vi "InjA-Image-FPGA.vi"() -> ()   [LabVIEW 2015]
uses:
  <vilib>/LabVIEW Targets/FPGA/cRIO/shared/nicrio_ModuleControls/nicrio_cRIO-9871_DataBitsEnum.ctl
  <vilib>/LabVIEW Targets/FPGA/cRIO/shared/nicrio_ModuleControls/nicrio_cRIO-9871_BaudRateEnum.ctl
  <vilib>/LabVIEW Targets/FPGA/cRIO/shared/nicrio_ModuleControls/nicrio_cRIO-9871_ParityEnum.ctl
  <vilib>/LabVIEW Targets/FPGA/cRIO/shared/nicrio_ModuleControls/nicrio_cRIO-9871_StopBitsEnum.ctl
  <vilib>/Platform/TimedLoop/XDataNode/timing_clust.ctl
  <vilib>/Platform/TimedLoop/XDataNode/nitl_modes.ctl
  <vilib>/Platform/TimedLoop/XDataNode/wakeup.ctl
  <vilib>/rvi/FXPMathLib/basic elements/FxpIntAccumulator/subVIs/nifxpmath_IntAccumulator_SimConfig.ctl
  <vilib>/rvi/Emulation/niFpgaGetClockAttributes.vi
  <vilib>/rvi/Emulation/niFpgaSctlEmulationGetInTimedLoop.vi
  <vilib>/rvi/Emulation/niFpgaEmulationReportErrorSimple.vi
  <vilib>/rvi/eio/common/nirviEmuTemplateMethod_errors.vi
  <vilib>/rvi/Emulation/niFpgaCriticalErrorInLSC.vi
  <vilib>/rvi/Analysis/common/codeGenErrors/XNode/niFpgaXNodeCodeGenErrorHandle.vi
  <vilib>/rvi/FXPMathLib/basic elements/FxpIntAccumulator/simVIs/DllFxpIntAccumulator_sub.vi
  <vilib>/rvi/eio/common/nirviEmuTemplatePropertySet_noerrors.vi
  <vilib>/eio/EIOMethodNode/EIOMethodNode.xnode
  <vilib>/eio/EIONode/EIONode.xnode
  <vilib>/rvi/Analysis/measure/dc-rms/XNode/niFpgaDC-RMS.xnode
  <vilib>/Platform/TimedLoop/XDataNode/XDataNode.xnode
  <vilib>/rvi/FXPMathLib/basic elements/FxpIntAccumulator/XNode/nifxpmath_IntAccumulator.xnode
  <vilib>/rvi/FXPMathLib/FxpMul/XNode/nifxpmath_Multiplier.xnode
  <vilib>/eio/EIOPropertyNode/EIOPropertyNode.xnode
  <vilib>/Platform/TimedLoop/XDataNode/XDNodeRunTimeDep.lvlib
  <vilib>/rvi/FXPMathLib/sim/FxpSim.dll
  <vilib>/rvi/eio/common/nirviEmuTemplatePropertyGet_errors.vi
  <vilib>/rvi/eio/common/nirviEmuTemplatePropertyGet_noerrors.vi
  <vilib>/rvi/eio/common/nirviEmuTemplatePropertySet_errors.vi
panel:
  in  "reset":bool
  out "Ion gauge 3":u8[](array[numeric])
  in  "cup set values":bool[](array[boolean])=[FALSE, FALSE, FALSE, FALSE]
  out "cup readbacks":bool[](array[boolean])
  out "1st stage temp(k)":u8[](array[numeric])
  out "2nd stage":u8[](array[numeric])
  out "Time on":u8[](array[numeric])
  out "Pump On":u8[](array[numeric])
  out "Ion gauge 4":u8[](array[numeric])
  out "Convectron 4":u8[](array[numeric])
  out "Convectron 3":u8[](array[numeric])
  out "Analog input":fxp<+/-,26,5>[](array[numeric]) format="%.23g"
  in  "analog output":fxp<+/-,64,32>[](array[numeric])=[0.0, 0.0, 0.0, 0.0, 0.0, 0.0, 0.0]
  in  "magnet ps":u8[](array[numeric])=[0, 0, 0, 0, 0, 0, 0, 0, 0, 0]
  out "error out":errorcluster
  out "magnet field":u8[](array[numeric])
  out "Timed Out":bool
  out "Data":u8
  # "skipped"
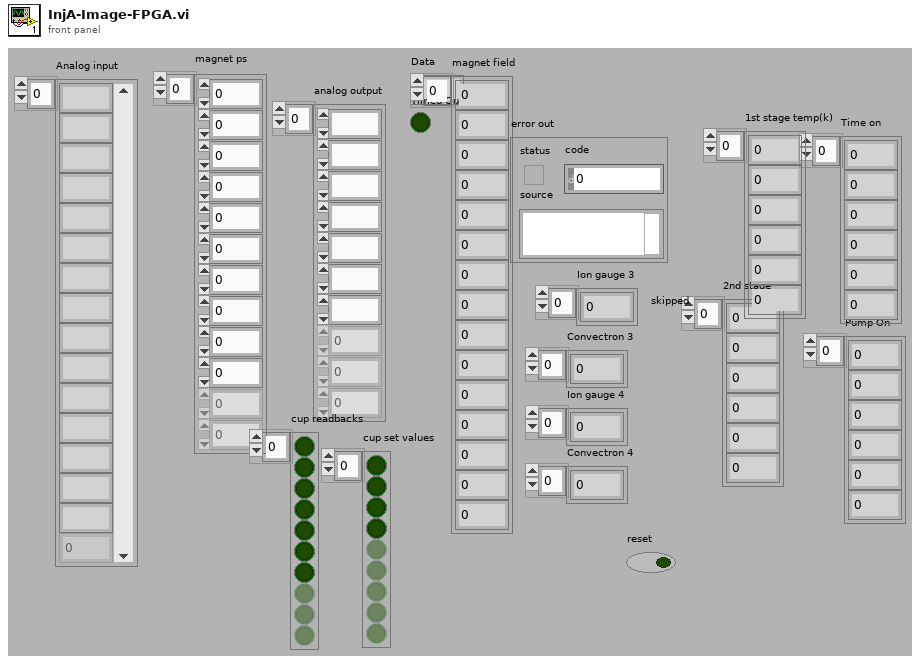
[diagram p1: front panel]
types:
  T1 = typedef "nicrio_cRIO-9871_BaudRateEnum.ctl" = enum16{"75 bps", "110 bps", "134 bps", "150 bps", "300 bps", "600 bps", "1200 bps", "1800 bps", "2400 bps", "4800 bps", "7200 bps", "9600 bps", "14.4 kbps", "19.2 kbps", "28.8 kbps", "38.4 kbps", "57.6 kbps", "115.2 kbps", "230.4 kbps", "460.8 kbps", "921.6 kbps"}
  T2 = typedef "nicrio_cRIO-9871_StopBitsEnum.ctl" = enum8{"1", "1.5", "2"}
  T3 = typedef "nicrio_cRIO-9871_ParityEnum.ctl" = enum8{"None", "Odd", "Even", "Mark", "Space"}
  T4 = typedef "nicrio_cRIO-9871_DataBitsEnum.ctl" = enum8{"5", "6", "7", "8"}
  T5 = typedef "XDNodeRunTimeDep.lvlib/timing_clust.ctl" = cluster{"Expected End [f-1]":u64, "Actual End [f-1]":u64, "Finished Late? [f-1]":bool, "Expected End [i-1]":u64, "Actual End [i-1]":u64, "Finished Late? [i-1]":bool, "Expected Start [i]":u64, "Actual Start [i]":u64, "Expected Start [f]":u64, "Actual Start [f]":u64, "Source Name":string, "Structure Name":string, "Period":i64, "Deadline":i64, "Offset":i64, "Start":i64, "Priority":i32, "Timeout":i32, "Mode":T6, "Wakeup Reason":T7, "Error":errorcluster, "Source Type":string, "Secondary Source Type":string, "Global End Time":u64, "Global Start Time":u64, "Frame Duration":u64, "Iteration Duration":u64, "Assigned CPU":i32, "I/O Scan Engine Mode":u32}
  T6 = typedef "XDNodeRunTimeDep.lvlib/nitl_modes.ctl" = enum32{"No Change", "Process missed periods, maintain original phase", "Discard missed periods, maintain original phase", "Process missed periods, ignore original phase", "Discard missed periods, ignore original phase"}
  T7 = typedef "XDNodeRunTimeDep.lvlib/wakeup.ctl" = enum32{"Normal", "Aborted", "Asynchronous wakeup", "Timing source error", "Timed loop error", "Timeout"}
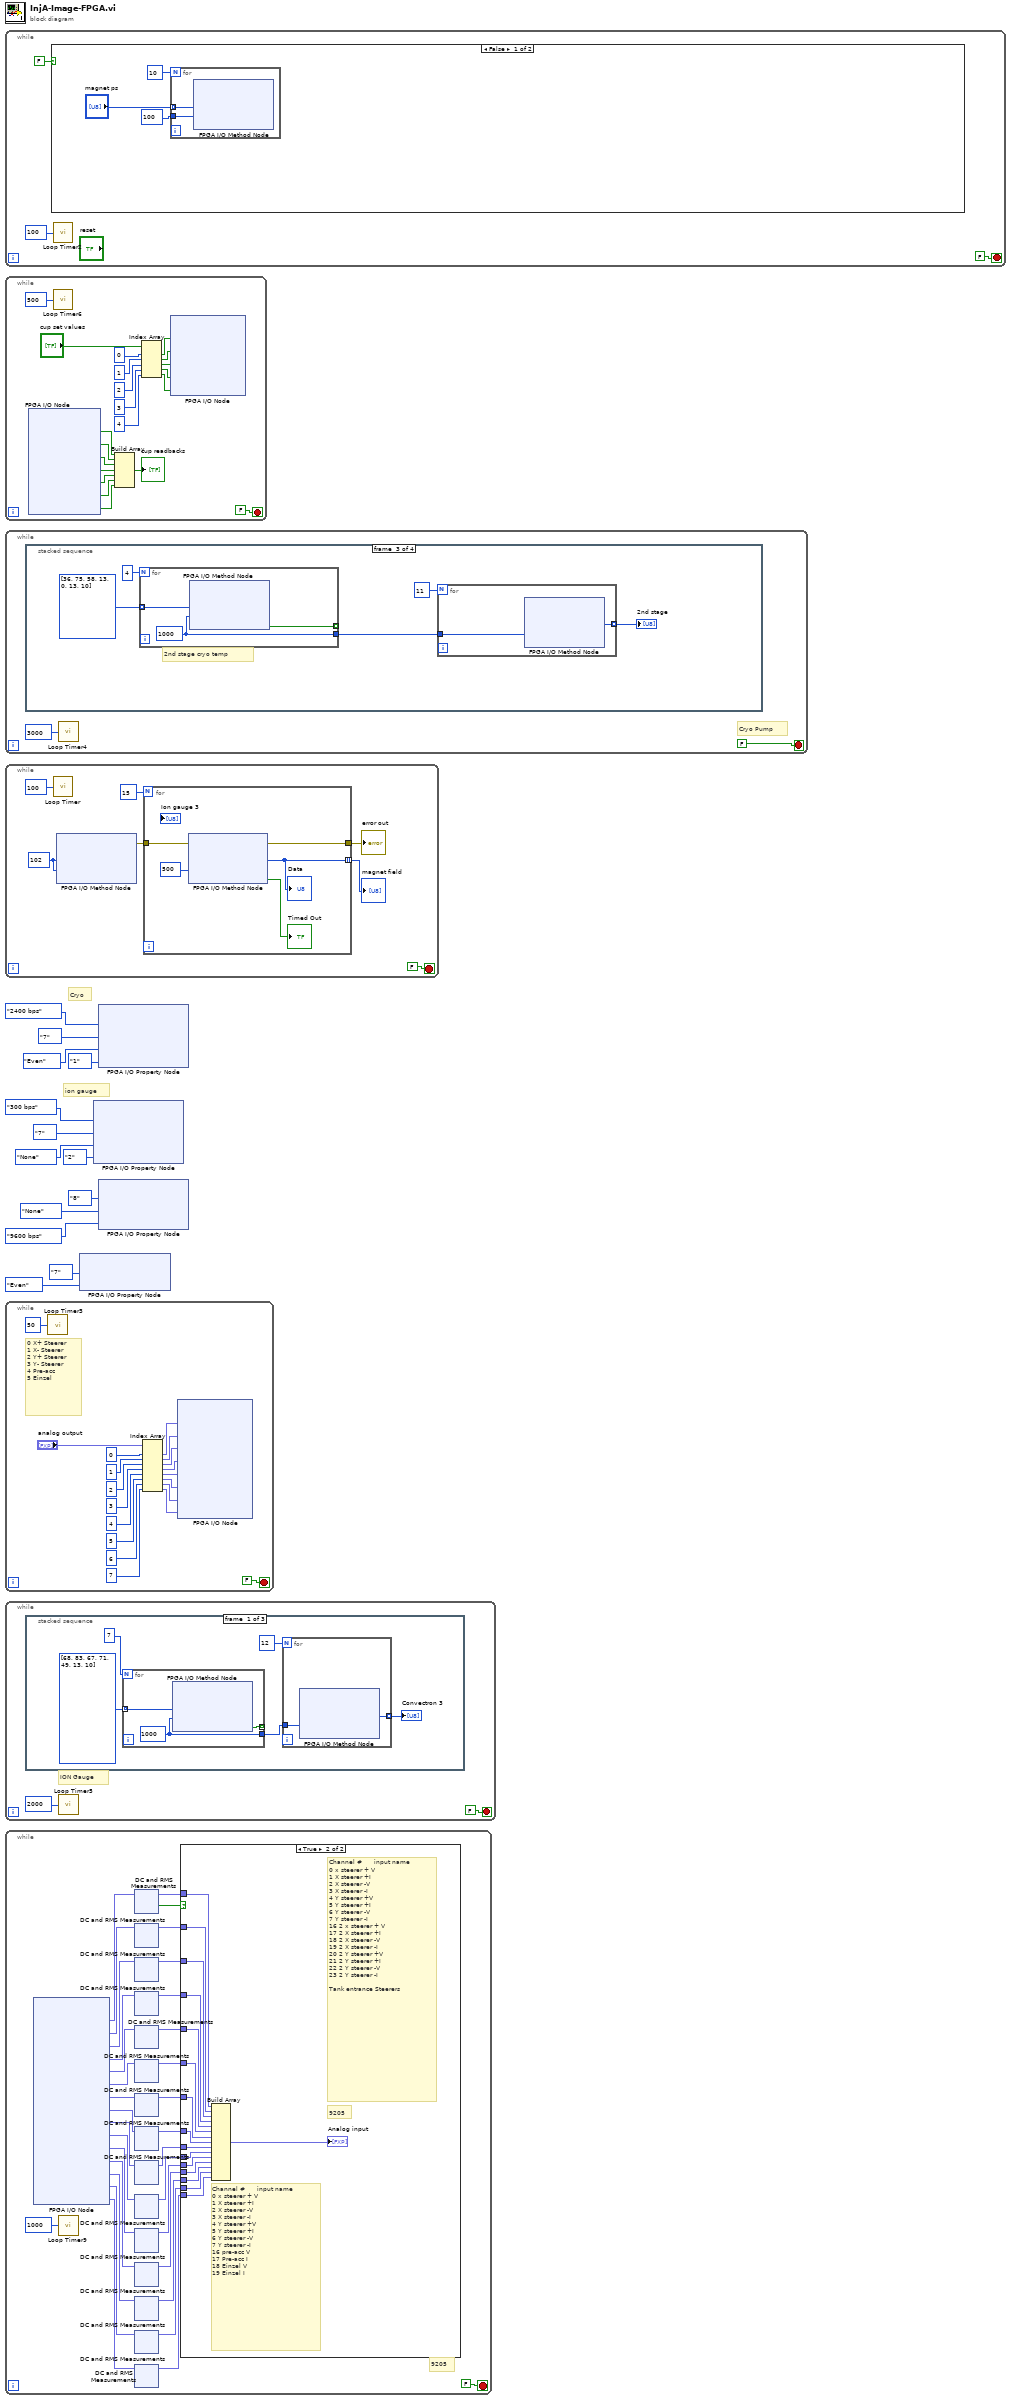
[diagram p0: block diagram]
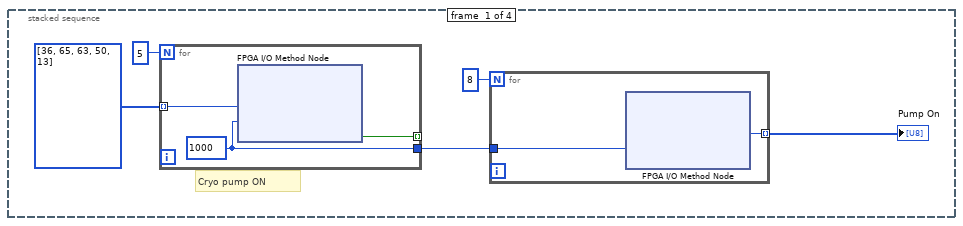
[diagram p3: hidden frame]
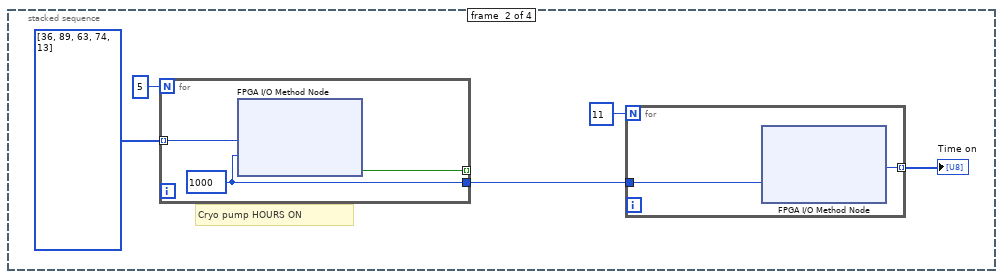
[diagram p4: hidden frame]
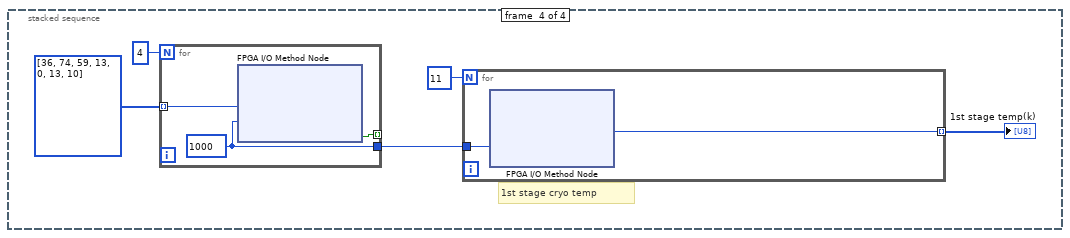
[diagram p5: hidden frame]
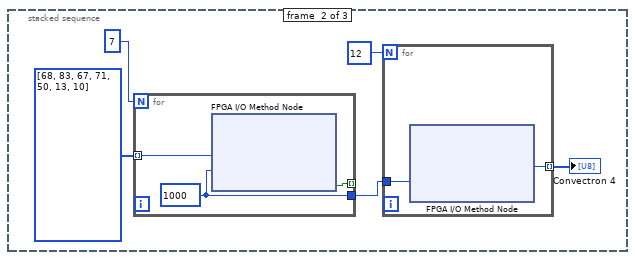
[diagram p6: hidden frame]
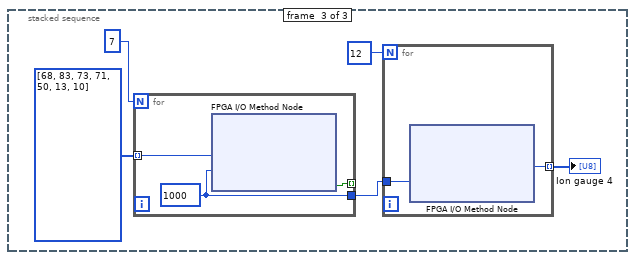
[diagram p7: hidden frame]
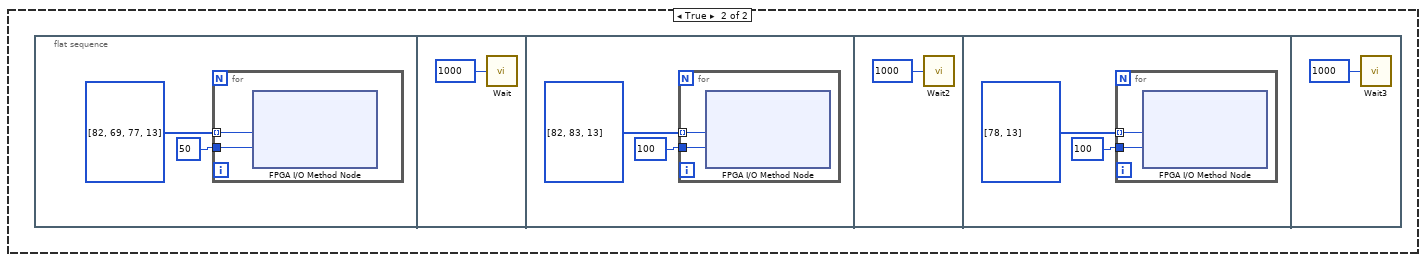
[diagram p8: hidden frame]
diagram:
  # "Cryo"
  # "ion gauge"
  n1 = while {
    stop <- FALSE stop-if-true
    n2 = case shown="False" FALSE {
      frame False {
        n3 = for {
          N: 10 -> [_]
          tunnel: 100 ("Timeout (ms)") -> [w21]
          tunnel: "magnet ps" -> [w20] mode=indexing
          n4 = xnode "FPGA I/O Method Node"("Data"=w20, "Timeout (ms)"=w21) -> ()  [unwired: 2 in, 3 out]
        }
      }
      frame True {
        n5 = flat-sequence {
          frame #0 {
            n6 = for {
              tunnel: 50 ("Timeout (ms)") -> [w25]
              tunnel: u8[] [82, 69, 77, 13] ("magnet ps") -> [w24] mode=indexing
              n7 = xnode "FPGA I/O Method Node"("Data"=w24, "Timeout (ms)"=w25) -> ()  [unwired: 2 in, 3 out]
            }
          }
          frame #1 {
            n8 = call "Wait"("Count(mSec)"=u32 1000) -> ()  [unwired: 1 out]
          }
          frame #2 {
            n9 = for {
              tunnel: 100 ("Timeout (ms)") -> [w30]
              tunnel: u8[] [82, 83, 13] ("magnet ps") -> [w29] mode=indexing
              n10 = xnode "FPGA I/O Method Node"("Data"=w29, "Timeout (ms)"=w30) -> ()  [unwired: 2 in, 3 out]
            }
          }
          frame #3 {
            n11 = call "Wait2"("Count(mSec)"=u32 1000) -> ()  [unwired: 1 out]
          }
          frame #4 {
            n12 = for {
              tunnel: 100 ("Timeout (ms)") -> [w35]
              tunnel: u8[] [78, 13] ("magnet ps") -> [w34] mode=indexing
              n13 = xnode "FPGA I/O Method Node"("Data"=w34, "Timeout (ms)"=w35) -> ()  [unwired: 2 in, 3 out]
            }
          }
          frame #5 {
            n14 = call "Wait3"("Count(mSec)"=u32 1000) -> ()  [unwired: 1 out]
          }
        }
      }
    }
    n15 = call "Loop Timer2"("Count(mSec)"=u32 100) -> ()  [unwired: 1 out]
  }
  n16 = while {
    stop <- FALSE stop-if-true
    n17 = xnode "FPGA I/O Node"() -> ("Mod4/DI0"=w56:bool, "Mod4/DI1"=w55:bool, "Mod4/DI2"=w54:bool, "Mod4/DI3"=w53:bool, "Mod4/DI4"=w39:bool, "Mod4/DI5"=w38:bool, "Mod4/DI6"=w37:bool)  [unwired: 7 in, 7 out]
    n18 = call "Loop Timer6"("Count(mSec)"=u32 500 ("Count(Ticks)")) -> ()  [unwired: 1 out]
    n19 = Build Array(w56, w55, w54, w53, w39, w38, w37) -> (→"cup readbacks":bool[])
    n20 = Index Array(array="cup set values", index #1=0 ("index"), index #2=1 ("index"), index #3=2 ("index"), index #4=3 ("index"), index #5=4 ("index")) -> (element #1=w45:bool, element #2=w44:bool, element #3=w43:bool, element #4=w42:bool, element #5=w41:bool)
    n21 = xnode "FPGA I/O Node"("Mod5/CH0"=w45, "Mod5/CH1"=w44, "Mod5/CH2"=w43, "Mod5/CH3"=w42, "Mod5/CH4"=w41) -> ()  [unwired: 5 in, 5 out]
  }
  n22 = while {
    stop <- FALSE stop-if-true
    # "Cryo Pump"
    n23 = stacked-sequence {
      frame #0 {
        # "Cryo pump ON"
        n24 = for {
          N: 5 -> [_]
          tunnel: [w69] -> w64
          tunnel: [w68] -> _ mode=indexing
          tunnel: u8[] [36, 65, 63, 50, 13] ("unsigned byte array") -> [w67] mode=indexing
          w69 = 1000 ("Timeout (ms)")
          n25 = xnode "FPGA I/O Method Node"("Data"=w67, "Timeout (ms)"=w69) -> ("Timed Out"=w68:bool)  [unwired: 1 in, 1 out]
        }
        n26 = for {
          N: 8 -> [_]
          tunnel: w64 -> [w66]
          tunnel: [w65] -> w60 mode=indexing
          n27 = xnode "FPGA I/O Method Node"("Timeout (ms)"=w66) -> ("Data"=w65:u8)  [unwired: 1 in, 2 out]
        }
        "Pump On" <- w60
      }
      frame #1 {
        # "Cryo pump HOURS ON"
        n28 = for {
          N: 5 -> [_]
          tunnel: [w79] -> w74
          tunnel: [w78] -> _ mode=indexing
          tunnel: u8[] [36, 89, 63, 74, 13] ("unsigned byte array") -> [w77] mode=indexing
          w79 = 1000 ("Timeout (ms)")
          n29 = xnode "FPGA I/O Method Node"("Data"=w77, "Timeout (ms)"=w79) -> ("Timed Out"=w78:bool)  [unwired: 1 in, 1 out]
        }
        n30 = for {
          N: 11 -> [_]
          tunnel: w74 -> [w76]
          tunnel: [w75] -> w70 mode=indexing
          n31 = xnode "FPGA I/O Method Node"("Timeout (ms)"=w76) -> ("Data"=w75:u8)  [unwired: 1 in, 2 out]
        }
        "Time on" <- w70
      }
      frame #2 {
        # "2nd stage cryo temp"
        n32 = for {
          N: 4 -> [_]
          tunnel: [w89] -> w84
          tunnel: [w88] -> _ mode=indexing
          tunnel: u8[] [36, 75, 58, 13, 0, 13, 10] ("unsigned byte array") -> [w87] mode=indexing
          w89 = 1000 ("Timeout (ms)")
          n33 = xnode "FPGA I/O Method Node"("Data"=w87, "Timeout (ms)"=w89) -> ("Timed Out"=w88:bool)  [unwired: 1 in, 1 out]
        }
        n34 = for {
          N: 11 -> [_]
          tunnel: w84 -> [w86]
          tunnel: [w85] -> w80 mode=indexing
          n35 = xnode "FPGA I/O Method Node"("Timeout (ms)"=w86) -> ("Data"=w85:u8)  [unwired: 1 in, 2 out]
        }
        "2nd stage" <- w80
      }
      frame #3 {
        # "1st stage cryo temp"
        n36 = for {
          N: 4 -> [_]
          tunnel: [w99] -> w94
          tunnel: [w98] -> _ mode=indexing
          tunnel: u8[] [36, 74, 59, 13, 0, 13, 10] ("unsigned byte array") -> [w97] mode=indexing
          w99 = 1000 ("Timeout (ms)")
          n37 = xnode "FPGA I/O Method Node"("Data"=w97, "Timeout (ms)"=w99) -> ("Timed Out"=w98:bool)  [unwired: 1 in, 1 out]
        }
        n38 = for {
          N: 11 -> [_]
          tunnel: w94 -> [w96]
          tunnel: [w95] -> w90 mode=indexing
          n39 = xnode "FPGA I/O Method Node"("Timeout (ms)"=w96) -> ("Data"=w95:u8)  [unwired: 1 in, 2 out]
        }
        "1st stage temp(k)" <- w90
      }
    }
    n40 = call "Loop Timer4"("Count(mSec)"=u32 3000 ("Count(Ticks)")) -> ()  [unwired: 1 out]
  }
  n41 = while {
    stop <- FALSE stop-if-true
    w103 = u8 102 ("Data")
    n42 = call "Loop Timer"("Count(mSec)"=u32 100) -> ()  [unwired: 1 out]
    n43 = xnode "FPGA I/O Method Node"("Data"=w103, "Timeout (ms)"=w103) -> ("error out"=w102:errorcluster)  [unwired: 2 in, 2 out]
    n44 = for {
      N: 15 ("Numeric 3") -> [_]
      tunnel: [w109] -> w104 mode=indexing
      tunnel: w102 -> [w108]
      tunnel: [w107] -> w101
      n45 = xnode "FPGA I/O Method Node"("error in"=w108, "Timeout (ms)"=500) -> ("error out"=w107:errorcluster, "Data"=w109:u8, "Timed Out"=→"Timed Out":bool)  [unwired: 1 in, 1 out]
      "Data" <- w109
    }
    "magnet field" <- w104
    "error out" <- w101
  }
  n46 = while {
    stop <- FALSE stop-if-true
    # "0 X+ Steerer\n1 X- Steerer\n2 Y+ Steerer\n3 Y- Steerer\n4 Pre-acc\n5 Einzel"
    n47 = call "Loop Timer3"("Count(mSec)"=u32 50) -> ()  [unwired: 1 out]
    n48 = Index Array(array="analog output", index #1=0 ("index"), index #2=1 ("index"), index #3=2 ("index"), index #4=3 ("index"), index #5=4 ("index"), index #6=5 ("index"), index #7=6 ("index"), index #8=7 ("index")) -> (element #1=w119:fxp<+/-,64,32>, element #2=w118:fxp<+/-,64,32>, element #3=w117:fxp<+/-,64,32>, element #4=w116:fxp<+/-,64,32>, element #5=w115:fxp<+/-,64,32>, element #6=w114:fxp<+/-,64,32>, element #7=w113:fxp<+/-,64,32>, element #8=w112:fxp<+/-,64,32>)
    n49 = xnode "FPGA I/O Node"("Mod1/AO0"=w119, "Mod1/AO1"=w118, "Mod1/AO2"=w117, "Mod1/AO3"=w116, "Mod1/AO4"=w115, "Mod1/AO5"=w114, "Mod1/AO6"=w113, "Mod1/AO7"=w112) -> ()  [unwired: 8 in, 8 out]
  }
  n50 = while {
    stop <- FALSE stop-if-true
    # "ION Gauge"
    n51 = stacked-sequence {
      frame #0 {
        n52 = for {
          N: 7 -> [_]
          tunnel: [w142] -> w137
          tunnel: [w141] -> _ mode=indexing
          tunnel: u8[] [68, 83, 67, 71, 49, 13, 10] ("unsigned byte array") -> [w140] mode=indexing
          w142 = 1000 ("Timeout (ms)")
          n53 = xnode "FPGA I/O Method Node"("Data"=w140, "Timeout (ms)"=w142) -> ("Timed Out"=w141:bool)  [unwired: 1 in, 1 out]
        }
        n54 = for {
          N: 12 -> [_]
          tunnel: w137 -> [w139]
          tunnel: [w138] -> w133 mode=indexing
          n55 = xnode "FPGA I/O Method Node"("Timeout (ms)"=w139) -> ("Data"=w138:u8)  [unwired: 1 in, 2 out]
        }
        "Convectron 3" <- w133
      }
      frame #1 {
        n56 = for {
          N: 7 -> [_]
          tunnel: [w152] -> w147
          tunnel: [w151] -> _ mode=indexing
          tunnel: u8[] [68, 83, 67, 71, 50, 13, 10] ("unsigned byte array") -> [w150] mode=indexing
          w152 = 1000 ("Timeout (ms)")
          n57 = xnode "FPGA I/O Method Node"("Data"=w150, "Timeout (ms)"=w152) -> ("Timed Out"=w151:bool)  [unwired: 1 in, 1 out]
        }
        n58 = for {
          N: 12 -> [_]
          tunnel: w147 -> [w149]
          tunnel: [w148] -> w143 mode=indexing
          n59 = xnode "FPGA I/O Method Node"("Timeout (ms)"=w149) -> ("Data"=w148:u8)  [unwired: 1 in, 2 out]
        }
        "Convectron 4" <- w143
      }
      frame #2 {
        n60 = for {
          N: 7 -> [_]
          tunnel: [w162] -> w157
          tunnel: [w161] -> _ mode=indexing
          tunnel: u8[] [68, 83, 73, 71, 50, 13, 10] ("unsigned byte array") -> [w160] mode=indexing
          w162 = 1000 ("Timeout (ms)")
          n61 = xnode "FPGA I/O Method Node"("Data"=w160, "Timeout (ms)"=w162) -> ("Timed Out"=w161:bool)  [unwired: 1 in, 1 out]
        }
        n62 = for {
          N: 12 -> [_]
          tunnel: w157 -> [w159]
          tunnel: [w158] -> w153 mode=indexing
          n63 = xnode "FPGA I/O Method Node"("Timeout (ms)"=w159) -> ("Data"=w158:u8)  [unwired: 1 in, 2 out]
        }
        "Ion gauge 4" <- w153
      }
    }
    n64 = call "Loop Timer5"("Count(mSec)"=u32 2000 ("Count(Ticks)")) -> ()  [unwired: 1 out]
  }
  n65 = while {
    stop <- FALSE stop-if-true
    # "9205"
    n66 = xnode "FPGA I/O Node"() -> ("Mod2/AI0"=w192:fxp<+/-,26,5>, "Mod2/AI1"=w190:fxp<+/-,26,5>, "Mod2/AI2"=w188:fxp<+/-,26,5>, "Mod2/AI3"=w186:fxp<+/-,26,5>, "Mod2/AI4"=w184:fxp<+/-,26,5>, "Mod2/AI5"=w182:fxp<+/-,26,5>, "Mod2/AI6"=w180:fxp<+/-,26,5>, "Mod2/AI7"=w178:fxp<+/-,26,5>, "Mod2/AI16"=w176:fxp<+/-,26,5>, "Mod2/AI17"=w174:fxp<+/-,26,5>, "Mod2/AI18"=w172:fxp<+/-,26,5>, "Mod2/AI19"=w170:fxp<+/-,26,5>, "Mod2/AI20"=w168:fxp<+/-,26,5>, "Mod2/AI21"=w166:fxp<+/-,26,5>, "Mod2/AI22"=w164:fxp<+/-,26,5>)  [unwired: 15 in, 15 out]
    n67 = call "Loop Timer9"("Count(Ticks)"=u32 1000) -> ()  [unwired: 1 out]
    n68 = xnode "DC and RMS Measurements"("input data"=w192) -> ("DC"=w191:fxp<+/-,26,5>, "output valid"=w193:bool)  [unwired: 1 in]
    n69 = xnode "DC and RMS Measurements"("input data"=w190) -> ("DC"=w189:fxp<+/-,26,5>)  [unwired: 1 in, 1 out]
    n70 = xnode "DC and RMS Measurements"("input data"=w188) -> ("DC"=w187:fxp<+/-,26,5>)  [unwired: 1 in, 1 out]
    n71 = xnode "DC and RMS Measurements"("input data"=w186) -> ("DC"=w185:fxp<+/-,26,5>)  [unwired: 1 in, 1 out]
    n72 = xnode "DC and RMS Measurements"("input data"=w184) -> ("DC"=w183:fxp<+/-,26,5>)  [unwired: 1 in, 1 out]
    n73 = xnode "DC and RMS Measurements"("input data"=w182) -> ("DC"=w181:fxp<+/-,26,5>)  [unwired: 1 in, 1 out]
    n74 = xnode "DC and RMS Measurements"("input data"=w180) -> ("DC"=w179:fxp<+/-,26,5>)  [unwired: 1 in, 1 out]
    n75 = xnode "DC and RMS Measurements"("input data"=w178) -> ("DC"=w177:fxp<+/-,26,5>)  [unwired: 1 in, 1 out]
    n76 = xnode "DC and RMS Measurements"("input data"=w176) -> ("DC"=w175:fxp<+/-,26,5>)  [unwired: 1 in, 1 out]
    n77 = xnode "DC and RMS Measurements"("input data"=w174) -> ("DC"=w173:fxp<+/-,26,5>)  [unwired: 1 in, 1 out]
    n78 = xnode "DC and RMS Measurements"("input data"=w172) -> ("DC"=w171:fxp<+/-,26,5>)  [unwired: 1 in, 1 out]
    n79 = xnode "DC and RMS Measurements"("input data"=w170) -> ("DC"=w169:fxp<+/-,26,5>)  [unwired: 1 in, 1 out]
    n80 = xnode "DC and RMS Measurements"("input data"=w168) -> ("DC"=w167:fxp<+/-,26,5>)  [unwired: 1 in, 1 out]
    n81 = xnode "DC and RMS Measurements"("input data"=w166) -> ("DC"=w165:fxp<+/-,26,5>)  [unwired: 1 in, 1 out]
    n82 = xnode "DC and RMS Measurements"("input data"=w164) -> ("DC"=w163:fxp<+/-,26,5>)  [unwired: 1 in, 1 out]
    n83 = case shown="True" w193 {
      tunnel: w191 -> [_ w371]
      tunnel: w189 -> [_ w370]
      tunnel: w187 -> [_ w369]
      tunnel: w185 -> [_ w368]
      tunnel: w183 -> [_ w367]
      tunnel: w181 -> [_ w366]
      tunnel: w179 -> [_ w365]
      tunnel: w177 -> [_ w364]
      tunnel: w175 -> [_ w363]
      tunnel: w173 -> [_ w362]
      tunnel: w171 -> [_ w361]
      tunnel: w169 -> [_ w360]
      tunnel: w167 -> [_ w359]
      tunnel: w165 -> [_ w358]
      tunnel: w163 -> [_ w357]
      frame False {
      }
      frame True {
        # "Channel #      input name\n0 x steerer + V\n1 X steerer +I\n2 X steerer -V\n3 X steerer -I\n4 Y steerer +V\n5 Y steerer +I\n6 Y steerer -V\n7 Y steerer -I\n16 pre-acc V\n17 Pre-acc I\n18 Einzel V\n19 Einzel I"
        # "Channel #      input name\n0 x steerer + V\n1 X steerer +I\n2 X steerer -V\n3 X steerer -I\n4 Y steerer +V\n5 Y steerer +I\n6 Y steerer -V\n7 Y steerer -I\n16 2 x steerer + V\n17 2 X steerer +I\n18 2 X steerer -V\n19 2 X steerer -I\n20 2 Y steerer +V\n21 2 Y steerer +I\n22 2 Y steerer -V\n23 2 Y steerer -I\n\nTank entrance Steerers"
        # "9205"
        n84 = Build Array(w371, w370, w369, w368, w367, w366, w365, w364, w363, w362, w361, w360, w359, w358, w357) -> (→"Analog input":fxp<+/-,26,5>[])
      }
    }
  }
  n85 = xnode "FPGA I/O Property Node"("Data Bits"=nicrio_cRIO-9871_DataBitsEnum."7", "Parity"=nicrio_cRIO-9871_ParityEnum."Even") -> ()  [unwired: 1 in, 1 out]
  n86 = xnode "FPGA I/O Property Node"("Baud Rate"=nicrio_cRIO-9871_BaudRateEnum."300 bps", "Data Bits"=nicrio_cRIO-9871_DataBitsEnum."7", "Parity"=nicrio_cRIO-9871_ParityEnum."None", "Stop Bits"=nicrio_cRIO-9871_StopBitsEnum."2") -> ()  [unwired: 1 in, 1 out]
  n87 = xnode "FPGA I/O Property Node"("Baud Rate"=nicrio_cRIO-9871_BaudRateEnum."2400 bps", "Data Bits"=nicrio_cRIO-9871_DataBitsEnum."7", "Parity"=nicrio_cRIO-9871_ParityEnum."Even", "Stop Bits"=nicrio_cRIO-9871_StopBitsEnum."1") -> ()  [unwired: 1 in, 1 out]
  n88 = xnode "FPGA I/O Property Node"("Data Bits"=nicrio_cRIO-9871_DataBitsEnum."8", "Parity"=nicrio_cRIO-9871_ParityEnum."None", "Baud Rate"=nicrio_cRIO-9871_BaudRateEnum."9600 bps") -> ()  [unwired: 1 in, 1 out]
